vi "Releaser.vi"(11 "Gear Manipulator.lvclass":refnum<class "Gear Manipulator.lvclass">) -> (3 "Gear Manipulator.lvclass":refnum<class "Gear Manipulator.lvclass">)   [LabVIEW 2016, in "Gear Manipulator.lvclass"]
uses:
  Gear Manipulator.lvclass
  Gear Manipulator.lvclass/Gear Manipulator.ctl
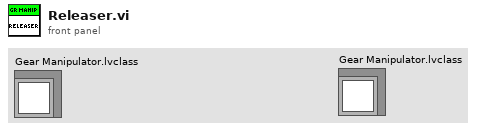
[diagram p1: front panel]
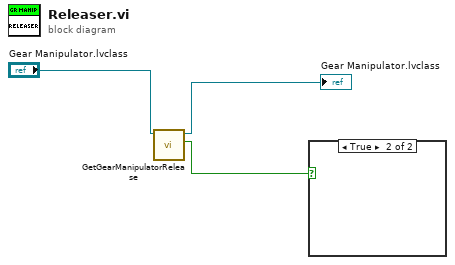
[diagram p0: block diagram]
diagram:
  n1 = call "GetGearManipulatorRelease.vi"("Gear Manipulator in"="Gear Manipulator.lvclass") -> ("Gear Manipulator Release"=w1:bool, "Gear Manipulator out"=→"Gear Manipulator.lvclass":refnum<class "Gear Manipulator.lvclass">)  [unwired: 9 in]
  n2 = case shown="True" w1 {
    frame False {
    }
    frame True {
    }
  }
